vi "4110_Current _Chan Config Dialog_RTM.vi"(8 "error in (no error)":errorcluster, 11 "CD PTR":T2 format="%.0x") -> (0 "error out":errorcluster, 1 "Channels to Add":u16[](array[numeric]), 2 "Voltage Limit (out)":dbl, 3 "Initial Current Value (out)":dbl, 4 "Remote Sense? Out":T1, 5 "Cancel (out)":bool)   [LabVIEW 2018, in "NI PXI-4110 Programmable Power Supply Custom Device.lvlib"]
uses:
  NI PXI-4110 Programmable Power Supply Custom Device.lvlib
  <vilib>/NI Veristand/Custom Device API/Custom Device Item Ref.ctl
  RemoteSense.ctl
  Power_Supply_In_Use.ctl
  4110_Global.vi
  <vilib>/NI Veristand/Custom Device API/Get Item Property (U16).vi
  <vilib>/NI Veristand/Custom Device API/Get Item Property (Boolean).vi
  <vilib>/NI VeriStand/Custom Device API/Custom Device API.lvlib
panel:
  in  "Remote Sense?":T1
  in  "Channel(s) to add":T3
  in  "Cancel":bool
  in  "OK Button":bool
  in  "Initial Current Value":dbl format="%.4f"
  in  "Voltage Limit":dbl
  # "Current Channels"
  # "Note: Channel 2 current\nvalues will be converted\nto negative values\nappropriately."
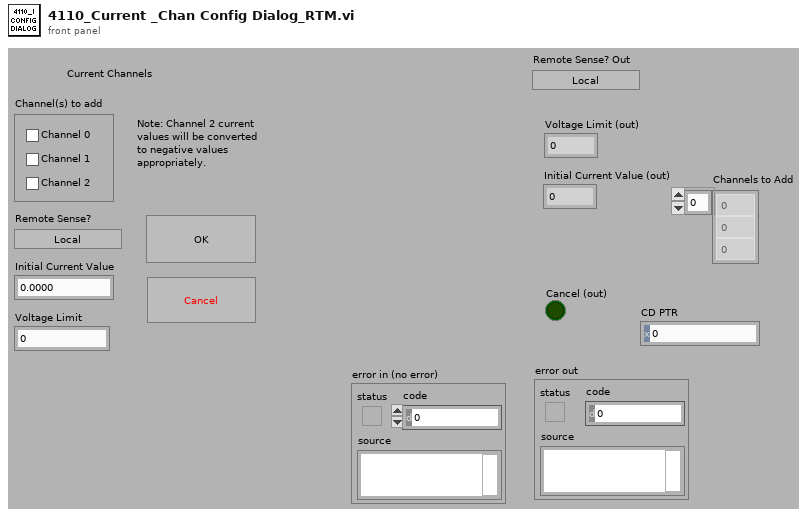
[diagram p1: front panel]
types:
  T1 = typedef "NI PXI-4110 Programmable Power Supply Custom Device.lvlib/RemoteSense.ctl" = bool
  T2 = typedef "Custom Device API.lvlib/Custom Device Item Ref.ctl" = u64
  T3 = cluster{"Channel 0":bool, "Channel 1":bool, "Channel 2":bool}
  T4 = enum8{"Enabled", "Disabled", "Disabled and Grayed Out"}
  T5 = typedef "NI PXI-4110 Programmable Power Supply Custom Device.lvlib/Power_Supply_In_Use.ctl" = enum16{"PXIe-4112", "PXI-4110"}
  T6 = cluster{"V_min":dbl, "V_max":dbl, "I_min":dbl, "I_max":dbl}
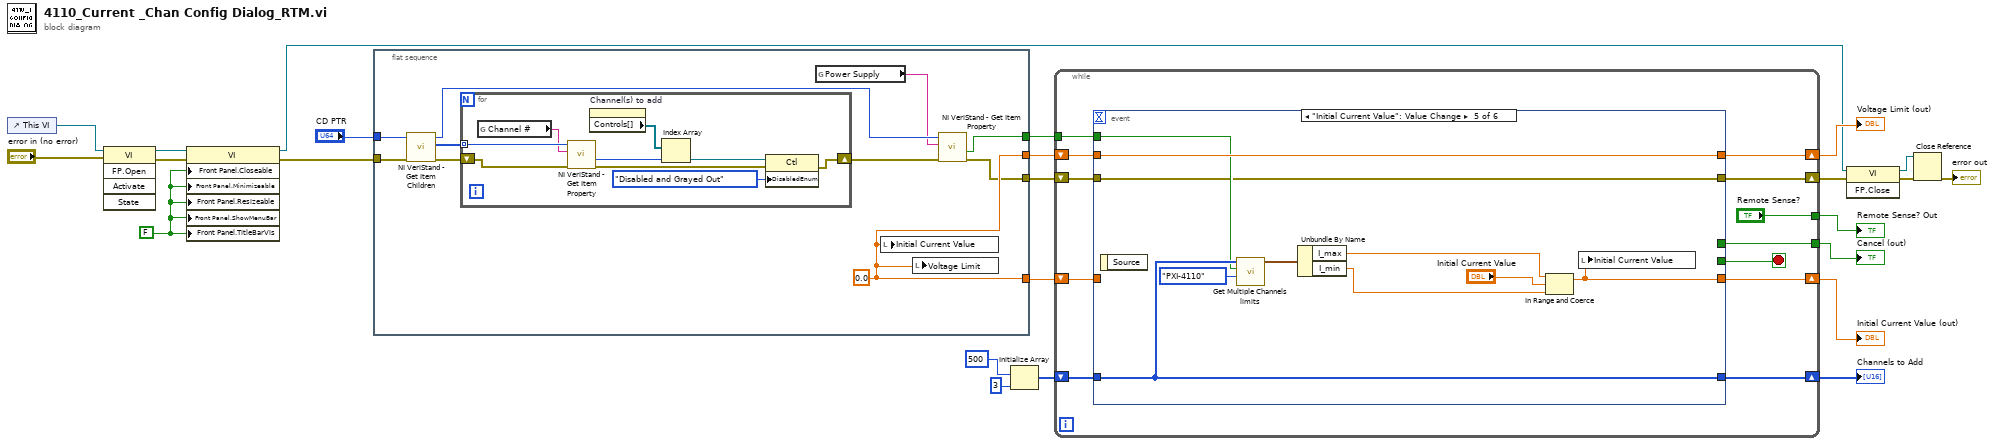
[diagram p0: block diagram]
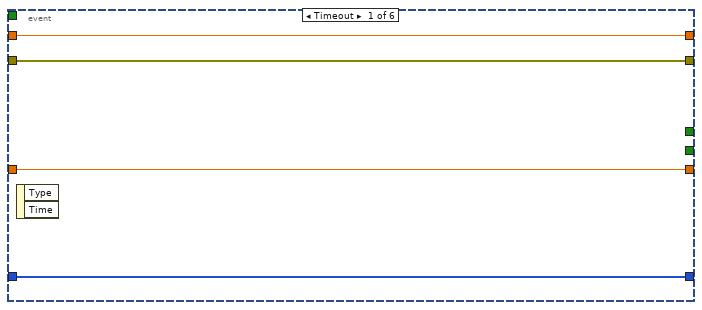
[diagram p2: hidden frame]
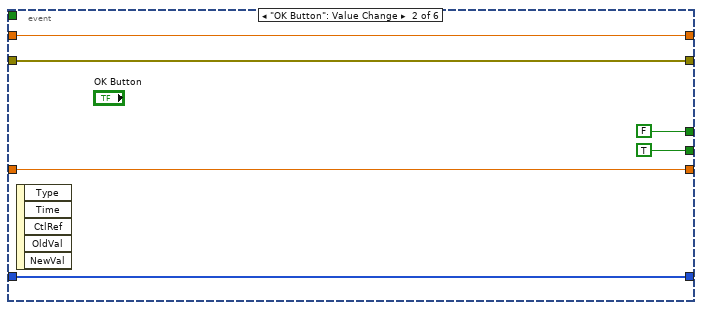
[diagram p3: hidden frame]
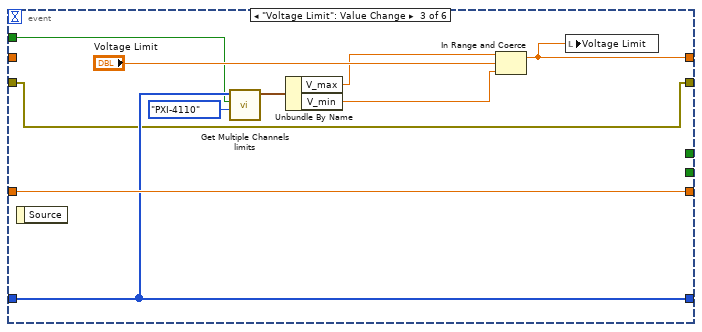
[diagram p4: hidden frame]
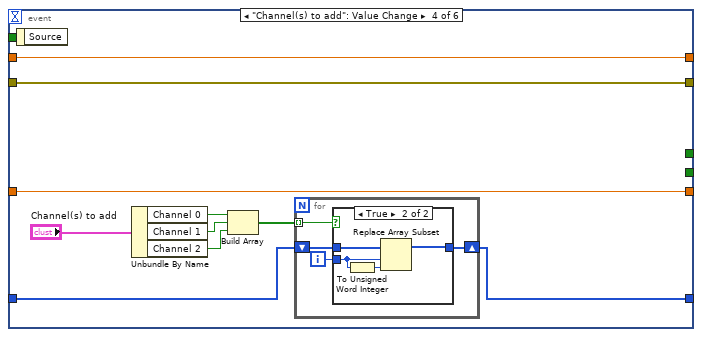
[diagram p5: hidden frame]
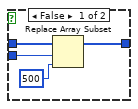
[diagram p6: hidden frame]
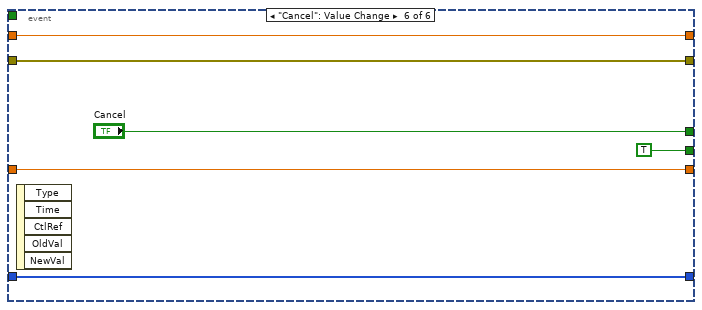
[diagram p7: hidden frame]
diagram:
  w11 = FALSE
  n1 = control-ref of="This VI"() -> (w8:refnum<vi>)
  n2 = invoke class="VI" method="FP.Open"(reference=w8, error in="error in (no error)") -> (reference out=w9:refnum<vi>, error out=w10:errorcluster)  [unwired: 3 in, 3 out]
  n3 = property class="VI"(reference=w9, error in=w10, "Front Panel.Closeable"=w11, "Front Panel.Minimizeable"=w11, "Front Panel.Resizeable"=w11, "Front Panel.ShowMenuBar"=w11, "Front Panel.TitleBarVis"=w11) -> (reference out=w5:refnum<vi>, error out=w6:errorcluster)
  n4 = flat-sequence {
    tunnel: [w25] -> w24
    tunnel: [w30] -> w20
    tunnel: [w30] -> w19
    tunnel: w6 -> [w34]
    tunnel: "CD PTR" -> [w33]
    tunnel: [w26] -> w17
    frame #0 {
      w30 = 0.0
      n5 = call <vilib>:"NI VeriStand - Get Item Children.vi"("error in (no error)"=w34, "Item Ref in"=w33) -> ("error out"=w31:errorcluster, "Child Refs"=w32:T2[], "Item Ref out"=w28:T2)  [unwired: 6 in, 1 out]
      n6 = for {
        tunnel: w32 -> [w43] mode=indexing
        shift-right: [w35] -> w29
        shift-left: w31 -> [w42]
        n7 = global read "4110_Global.vi" "Channel #"() -> (w41:string)
        n8 = call-poly <vilib>:"NI VeriStand - Get Item Property.vi"("error in (no error)"=w42, "Property Name"=w41, "Item Ref in"=w43) -> ("error out"=w36:errorcluster, "Value"=w37:u16)  [unwired: 5 in, 2 out]
        n9 = property on="Channel(s) to add" class="Clust (strict)"() -> ("Controls[]"=w39:refnum<vi>[])  [unwired: 2 in, 2 out]
        n10 = Index Array(array=w39, index=w37) -> (element=w40:refnum<vi>)
        n11 = property class="Ctl"(reference=w40, error in=w36, "DisabledEnum"=T4."Disabled and Grayed Out" ("Disabled")) -> (error out=w35:errorcluster)  [unwired: 1 out]
      }
      n12 = global read "4110_Global.vi" "Power Supply"() -> (w27:string)
      n13 = local write "Initial Current Value"(w30) -> ()
      n14 = local write "Voltage Limit"(w30) -> ()
      n15 = call-poly <vilib>:"NI VeriStand - Get Item Property.vi"("error in (no error)"=w29, "Property Name"=w27, "Item Ref in"=w28) -> ("error out"=w25:errorcluster, "Value"=w26:bool)  [unwired: 5 in, 2 out]
    }
  }
  n16 = Initialize Array(u16 500 ("element"), 3 ("dimension size")) -> (w14:u16[])
  n17 = while {
    tunnel: [w51] -> w21
    shift-right: [w54] -> w4
    shift-left: w24 -> [w55]
    shift-right: [w53] -> w23
    shift-left: w20 -> [w49]
    shift-right: [w52] -> w22
    shift-left: w19 -> [w48]
    tunnel: w17 -> [w47]
    shift-right: [w45] -> w13
    shift-left: w14 -> [w46]
    tunnel: ["Remote Sense?"] -> w12
    stop <- w50 stop-if-true
    n18 = event shown="[4] \"Initial Current Value\": Value Change" {
      selector: _ -> [_ _ _ _ _ _]
      dyn-events: _ -> [_ _ _ _ _ _]
      timeout: _ -> [_ _ _ _ _ _]
      tunnel: [w59 w62 w75 w85 w106 w111] -> w53
      tunnel: [w58 w61 w73 w84 w105 w110] -> w52
      tunnel: w55 -> [w56 w65 w66 w76 w98 w108]
      tunnel: [w56 w65 w66 w76 w98 w108] -> w54
      tunnel: [_ FALSE ("Cancel") _ _ _ "Cancel"] -> w51
      tunnel: [_ TRUE ("Cancel") _ _ _ TRUE ("Cancel")] -> w50
      tunnel: w49 -> [w59 w62 w75 w85 _ w111]
      tunnel: w48 -> [w58 w61 _ w84 w105 w110]
      tunnel: w47 -> [_ _ w71 _ w103 _]
      tunnel: w46 -> [w57 w60 w72 w78 w104 w109]
      tunnel: [w57 w60 w72 w77 w104 w109] -> w45
      event Timeout {
        n19 = event-data() -> ()  [unwired: 1 in, 2 out]
      }
      event "OK Button": Value Change {
        n20 = event-data() -> ()  [unwired: 1 in, 5 out]
      }
      event "Voltage Limit": Value Change {
        n21 = event-data() -> ()  [unwired: 1 in, 1 out]
        n22 = call "Get Multiple Channels limits.vi"("Power Supply In Use"=Power_Supply_In_Use."PXI-4110", "External Supply?"=w71, "Channels"=w72) -> ("output cluster"=w69:T6)  [unwired: 7 in, 1 out]
        n23 = Unbundle By Name(w69) -> ("V_max"=w68:dbl, "V_min"=w67:dbl)
        n24 = In Range and Coerce(upper limit=w68, x="Voltage Limit", lower limit=w67) -> (coerced(x)=w73:dbl)  [unwired: 1 out]
        n25 = local write "Voltage Limit"(w73) -> ()
      }
      event "Channel(s) to add": Value Change {
        n26 = event-data() -> ()  [unwired: 1 in, 1 out]
        n27 = Unbundle By Name("Channel(s) to add") -> ("Channel 0"=w82:bool, "Channel 1"=w81:bool, "Channel 2"=w80:bool)
        n28 = Build Array(w82, w81, w80) -> (w79:bool[])
        n29 = for {
          tunnel: w79 -> [w89] mode=indexing
          shift-right: [w86] -> w77
          shift-left: w78 -> [w88]
          i -> [w87]
          n30 = case shown="True" w89 {
            tunnel: w88 -> [w92 w97]
            tunnel: w87 -> [w93 w95]
            tunnel: [w90 w96] -> w86
            frame False {
              n31 = Replace Array Subset(array=w92, new element=u16 500 ("new element/subarray"), index=w93) -> (w90:u16[])
            }
            frame True {
              n32 = To Unsigned Word Integer(number=w95) -> (unsigned 16bit integer=w94:u16)
              n33 = Replace Array Subset(array=w97, new element=w94, index=w95) -> (w96:u16[])
            }
          }
        }
      }
      event "Initial Current Value": Value Change {
        n34 = event-data() -> ()  [unwired: 1 in, 1 out]
        n35 = call "Get Multiple Channels limits.vi"("Power Supply In Use"=Power_Supply_In_Use."PXI-4110", "External Supply?"=w103, "Channels"=w104) -> ("output cluster"=w101:T6)  [unwired: 7 in, 1 out]
        n36 = Unbundle By Name(w101) -> ("I_max"=w100:dbl, "I_min"=w99:dbl)
        n37 = In Range and Coerce(upper limit=w100, x="Initial Current Value", lower limit=w99) -> (coerced(x)=w106:dbl)  [unwired: 1 out]
        n38 = local write "Initial Current Value"(w106) -> ()
      }
      event "Cancel": Value Change {
        n39 = event-data() -> ()  [unwired: 1 in, 5 out]
      }
    }
  }
  "Initial Current Value (out)" <- w23
  "Voltage Limit (out)" <- w22
  "Cancel (out)" <- w21
  "Channels to Add" <- w13
  "Remote Sense? Out" <- w12
  n40 = invoke class="VI" method="FP.Close"(reference=w5, error in=w4) -> (reference out=w2:refnum<vi>, error out=w3:errorcluster)  [unwired: 1 in, 1 out]
  n41 = Close Reference(reference=w2, error in (no error)=w3) -> (error out=→"error out":errorcluster)
